vi "SIMULAREA EFECTELOR GRAFICE.vi"() -> ()   [LabVIEW 2025]
panel:
  in  "VITEZA EFECT":dbl(knob) scale=200.0..2000.0
  in  "ON / OFF":bool
  in  "SELECTIE CADRU":T1(ring)
  out "v 1\nV 8":bool[][](array[boolean])
  out "v 1\nV 7":bool[][](array[boolean])
  out "v 1\nV 6":bool[][](array[boolean])
  out "v 1\nV 5":bool[][](array[boolean])
  out "v 1\nV 4":bool[][](array[boolean])
  out "v 1\nV 3":bool[][](array[boolean])
  out "v 1\nV 2":bool[][](array[boolean])
  out "v 1\nV 1":bool[][](array[boolean])
  in  "MAIN":bool[][](array[boolean])
  in  "stop":bool
  # "SIMULAREA EFECTELOR GRAFICE LA NIVELUL MATRICEI CU 8X8 LEDURI CONECTATA LA ARDUINO"
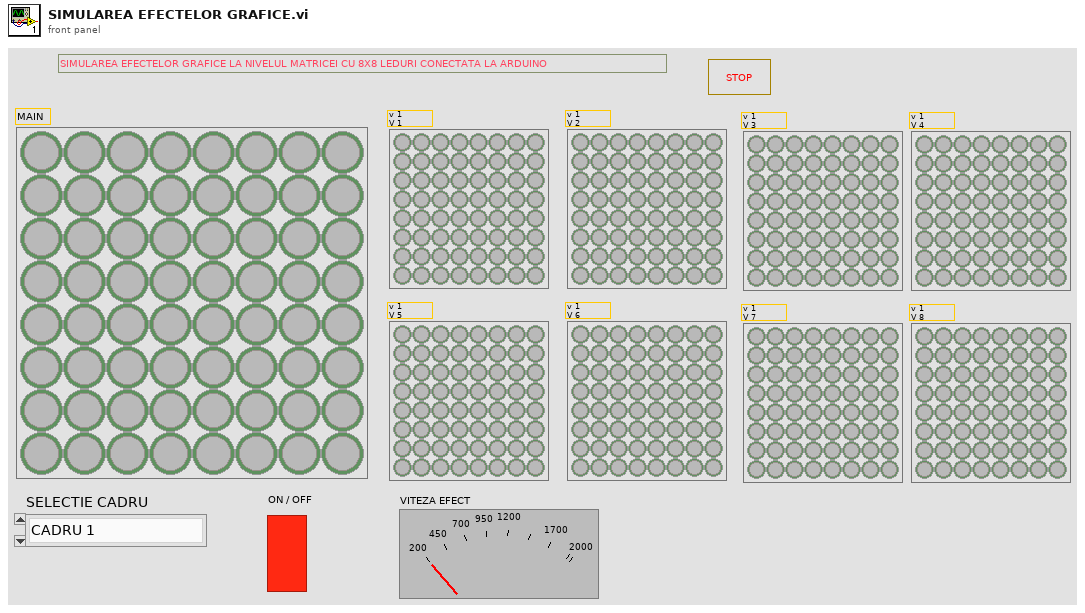
[diagram p1: front panel]
types:
  T1 = enum16{"CADRU 1", "CADRU 2", "CADRU 3", "CADRU 4", "CADRU 5", "CADRU 6", "CADRU 7", "CADRU 8"}
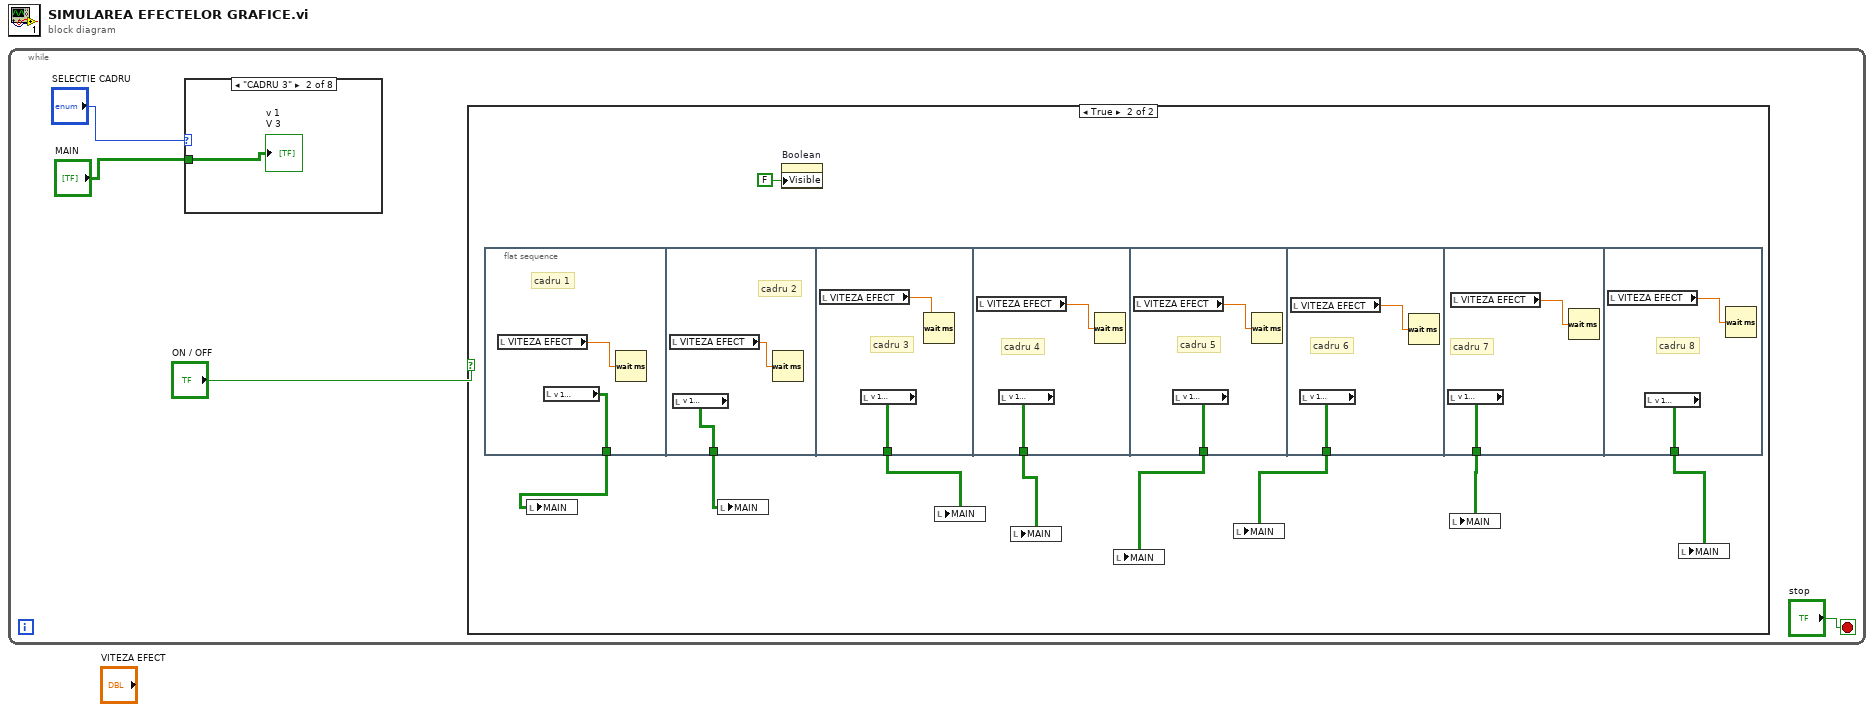
[diagram p0: block diagram]
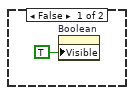
[diagram p2: hidden frame]
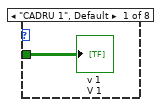
[diagram p3: hidden frame]
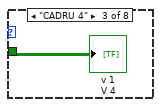
[diagram p4: hidden frame]
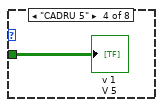
[diagram p5: hidden frame]
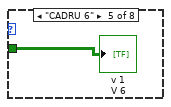
[diagram p6: hidden frame]
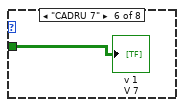
[diagram p7: hidden frame]
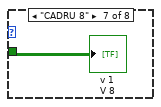
[diagram p8: hidden frame]
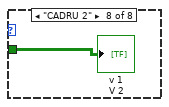
[diagram p9: hidden frame]
diagram:
  n1 = while {
    stop <- "stop" stop-if-true
    n2 = case shown="\"CADRU 3\"" "SELECTIE CADRU" {
      tunnel: "MAIN" -> [w31 w32 w33 w34 w35 w36 w37 w38]
      frame "CADRU 1", Default {
        "v 1\nV 1" <- w31
      }
      frame "CADRU 3" {
        "v 1\nV 3" <- w32
      }
      frame "CADRU 4" {
        "v 1\nV 4" <- w33
      }
      frame "CADRU 5" {
        "v 1\nV 5" <- w34
      }
      frame "CADRU 6" {
        "v 1\nV 6" <- w35
      }
      frame "CADRU 7" {
        "v 1\nV 7" <- w36
      }
      frame "CADRU 8" {
        "v 1\nV 8" <- w37
      }
      frame "CADRU 2" {
        "v 1\nV 2" <- w38
      }
    }
    n3 = case shown="True" "ON / OFF" {
      frame False {
        n4 = property on="Boolean" class="Bool (strict)"("Visible"=TRUE) -> ()  [unwired: 2 in, 2 out]
      }
      frame True {
        n5 = flat-sequence {
          tunnel: [w15] -> w7
          tunnel: [w17] -> w8
          tunnel: [w20] -> w14
          tunnel: [w22] -> w13
          tunnel: [w24] -> w12
          tunnel: [w26] -> w11
          tunnel: [w28] -> w10
          tunnel: [w30] -> w9
          frame #0 {
            # "cadru 1"
            n6 = local read "VITEZA EFECT"() -> (w16:dbl)
            n7 = local read "v 1\nV 1"() -> (w15:bool[][])
            n8 = Wait (ms)(milliseconds to wait=w16) -> ()  [unwired: 1 out]
          }
          frame #1 {
            # "cadru 2"
            n9 = local read "VITEZA EFECT"() -> (w18:dbl)
            n10 = local read "v 1\nV 2"() -> (w17:bool[][])
            n11 = Wait (ms)(milliseconds to wait=w18) -> ()  [unwired: 1 out]
          }
          frame #2 {
            # "cadru 3"
            n12 = local read "VITEZA EFECT"() -> (w19:dbl)
            n13 = local read "v 1\nV 3"() -> (w20:bool[][])
            n14 = Wait (ms)(milliseconds to wait=w19) -> ()  [unwired: 1 out]
          }
          frame #3 {
            # "cadru 4"
            n15 = local read "VITEZA EFECT"() -> (w21:dbl)
            n16 = local read "v 1\nV 4"() -> (w22:bool[][])
            n17 = Wait (ms)(milliseconds to wait=w21) -> ()  [unwired: 1 out]
          }
          frame #4 {
            # "cadru 5"
            n18 = local read "VITEZA EFECT"() -> (w23:dbl)
            n19 = local read "v 1\nV 5"() -> (w24:bool[][])
            n20 = Wait (ms)(milliseconds to wait=w23) -> ()  [unwired: 1 out]
          }
          frame #5 {
            # "cadru 6"
            n21 = local read "VITEZA EFECT"() -> (w25:dbl)
            n22 = local read "v 1\nV 6"() -> (w26:bool[][])
            n23 = Wait (ms)(milliseconds to wait=w25) -> ()  [unwired: 1 out]
          }
          frame #6 {
            # "cadru 7"
            n24 = local read "v 1\nV 7"() -> (w28:bool[][])
            n25 = local read "VITEZA EFECT"() -> (w27:dbl)
            n26 = Wait (ms)(milliseconds to wait=w27) -> ()  [unwired: 1 out]
          }
          frame #7 {
            # "cadru 8"
            n27 = local read "VITEZA EFECT"() -> (w29:dbl)
            n28 = local read "v 1\nV 8"() -> (w30:bool[][])
            n29 = Wait (ms)(milliseconds to wait=w29) -> ()  [unwired: 1 out]
          }
        }
        n30 = local write "MAIN"(w7) -> ()
        n31 = local write "MAIN"(w8) -> ()
        n32 = property on="Boolean" class="Bool (strict)"("Visible"=FALSE) -> ()  [unwired: 2 in, 2 out]
        n33 = local write "MAIN"(w14) -> ()
        n34 = local write "MAIN"(w13) -> ()
        n35 = local write "MAIN"(w12) -> ()
        n36 = local write "MAIN"(w11) -> ()
        n37 = local write "MAIN"(w10) -> ()
        n38 = local write "MAIN"(w9) -> ()
      }
    }
  }
